vi "metin belgesine veri yazdırma.vi"() -> ()   [LabVIEW 2014]
panel:
  in  "Path":path
  in  "okul no":string
  in  "Soyad":string
  in  "Ad":string
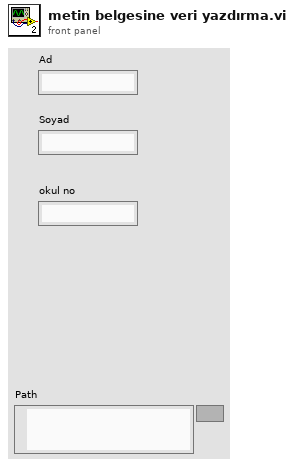
[diagram p1: front panel]
types:
  T1 = enum16{"open", "replace", "create", "open or create", "replace or create", "replace or create with confirmation"}
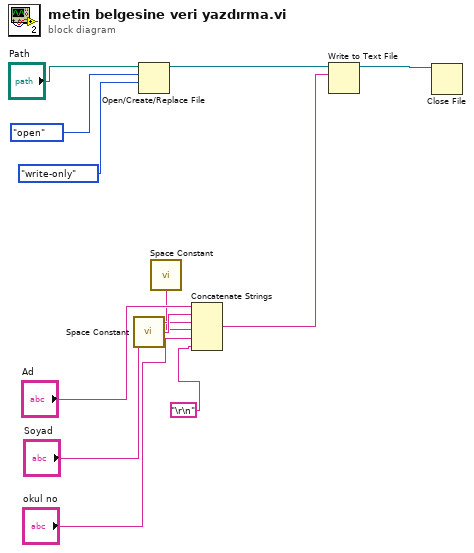
[diagram p0: block diagram]
diagram:
  n1 = call <vilib>:"Space Constant.vi"() -> ("String"=w5:string)
  n2 = Open/Create/Replace File(file path (use dialog)="Path", operation (0:open)=T1."open", access (0:read/write)=enum16{"read/write", "read-only", "write-only"}."write-only") -> (refnum out=w9:refnum<file>)  [unwired: 3 in, 2 out]
  n3 = call <vilib>:"Space Constant.vi"() -> ("String"=w3:string)
  n4 = Concatenate Strings("Ad", w5, "Soyad", w3, "okul no", "\r\n") -> (w6:string)
  n5 = Write to Text File(file (use dialog)=w9, text=w6) -> (refnum out=w8:refnum<file>)  [unwired: 2 in, 2 out]
  n6 = Close File(refnum=w8) -> ()  [unwired: 1 in, 2 out]
